vi "OpenBoard.vi"(8 "error in (no error)":errorcluster, 10 "Board Address":u8 max=31, 11 "VISA resource name":refnum<visa-resource-name>) -> (0 "error out":errorcluster, 3 "BoardHandle":T1)   [LabVIEW 2018, in "CAEN PSM.lvlib"]
doc: "This function allows to open the device. Therefore, call this VI after calling Initialize.vi. You can need to call this function more times if you use several boards in daisy chain."
uses:
  CAEN PSM.lvlib
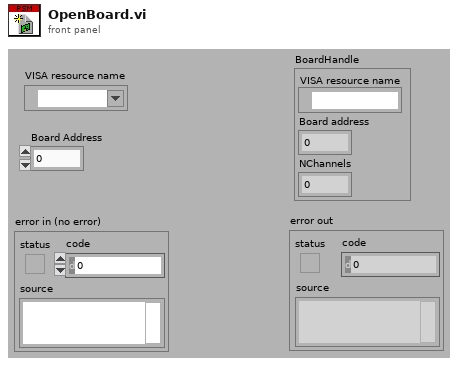
[diagram p1: front panel]
types:
  T1 = cluster{"VISA resource name":refnum<visa-resource-name>, "Board address":u8, "NChannels":u8}
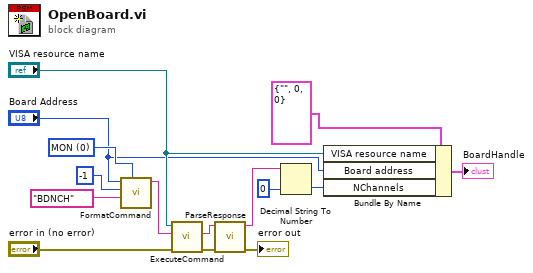
[diagram p0: block diagram]
diagram:
  w13 = u8 0 items=["MON", "SET"] ("CMD")
  n1 = call "FormatCommand.vi"("CMD (MON)"=w13, "PAR"="BDNCH", "CH"=i8 -1, "BD (0)"="Board Address") -> ("cmd"=w2:string)  [unwired: 7 in]
  n2 = call "ExecuteCommand.vi"("error in (no error)"="error in (no error)", "Command"=w2, "VISA resource name"="VISA resource name") -> ("error out"=w3:errorcluster, "Response"=w4:string)  [unwired: 6 in, 1 out]
  n3 = call "ParseResponse.vi"("error in (no error)"=w3, "Response"=w4) -> ("error out"=→"error out":errorcluster, "val"=w1:string)  [unwired: 6 in, 2 out]
  n4 = Decimal String To Number(string=w1, default (0L)=u8 0 ("default (0 I32)")) -> (number=w9:u8)  [unwired: 1 in, 1 out]
  n5 = Bundle By Name(cluster=T1 {"VISA resource name"="", "Board address"=0, "NChannels"=0} ("BoardHandle"), "VISA resource name"="VISA resource name", "Board address"="Board Address", "NChannels"=w9) -> (→"BoardHandle":T1)
